vi "TDMS Advanced Append Multiple Headers.vi"   [LabVIEW 2023]
doc: "This example demonstrates how to append new header and raw data to an existing .tdms file using the Advanced TDMS VIs and functions. You can use the TDMS Advanced Asynchronous Read function to read the data from the .tdms file."
uses:
  <vilib>/Utility/TDMS File Viewer/NI_TDMS File Viewer.lvlib
panel:
  # "Overview: Demonstrates the use of the Advanced TDMS functions to append data with headers to a .tdms file.\nInstructions:\n1. Make sure you have already run TDMS Advanced Asynchronous Write.vi.\n2. Run this VI.\n3. Delete the TDMS file (located at [LabVIEW Data]\\Example TDMS Advanced Asynchronous Write.tdms) when you are done."
types:
  T1 = enum16{"open", "open or create", "create or replace", "create", "open (read-only)"}
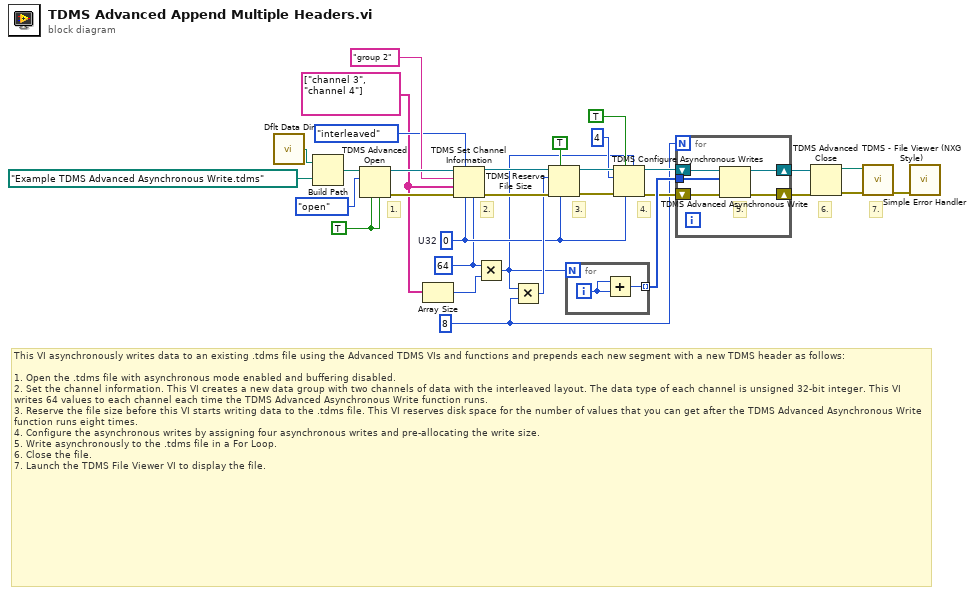
[diagram p0: block diagram]
diagram:
  w17 = TRUE ("enable asynchronous? (T)")
  w5 = 8 ("y")
  w3 = u32 64 ("samples per channel")
  w9 = u32 0  # U32
  w4 = string[] ["channel 3", "channel 4"] ("channel name(s)")
  # "4."
  # "This VI asynchronously writes data to an existing .tdms file using the Advanced TDMS VIs and functions and prepends each new segment with a new TDMS header as follows:\n\n1. Open the .tdms file with asynchronous mode enabled and buffering disabled.\n2. Set the channel information. This VI creates a new data group with two channels of data with the interleaved layout. The data type of each channel is unsigned 32-bit integer. This VI writes 64 values to each channel each time the TDMS Advanced Asynchronous Write function runs.\n3. Reserve the file size before this VI starts writing data to the .tdms file. This VI reserves disk space for the number of values that you can get after the TDMS Advanced Asynchronous Write function runs eight times.\n4. Configure the asynchronous writes by assigning four asynchronous writes and pre-allocating the write size.\n5. Write asynchronously to the .tdms file in a For Loop.\n6. Close the file.\n7. Launch the TDMS File Viewer VI to display the file."
  # "7."
  # "1."
  # "6."
  # "3."
  # "2."
  n1 = call <vilib>:"Dflt Data Dir.vi"() -> ("App:Default Data Directory"=w26:path)
  n2 = Build Path(base path=w26, name or relative path=path "Example TDMS Advanced Asynchronous Write.tdms") -> (appended path=w30:path)
  n3 = TDMS Advanced Open(4:w17, 6:w17, 10:T1."open" ("operation (0:open)"), 11:w30) -> (0:w28:errorcluster, 3:w27:refnum<k34>)  [unwired: 1 in, 1 out]
  n4 = Array Size(array=w4) -> (size(s)=w2:i32)
  n5 = TDMS Set Channel Information(4:w3, 6:w9, 7:enum16{"non-interleaved", "interleaved"}."interleaved" ("data layout (0:non-interleaved)"), 8:w28, 9:w4, 10:"group 2" ("group name (Untitled)"), 11:w27) -> (0:w20:errorcluster, 3:w19:refnum<k34>)
  n6 = Multiply(x=w3, y=w2) -> (x*y=w1:u32)
  n7 = Multiply(x=w1, y=w5) -> (x*y=w18:u32)
  n8 = TDMS Reserve File Size(6:w9, 7:TRUE ("append? (T)"), 8:w20, 10:w18, 11:w19) -> (0:w14:errorcluster, 3:w13:refnum<k34>)
  n9 = for {
    N: w1 -> [_]
    tunnel: [w32] -> w23 mode=indexing
    i -> [w33]
    n10 = Add(x=w33, y=w33) -> (x+y=w32:i32)
  }
  n11 = TDMS Configure Asynchronous Writes(5:w1, 6:w9, 7:TRUE ("pre-allocate? (F)"), 8:w14, 10:u32 4 ("number of buffers (4)"), 11:w13) -> (0:w11:errorcluster, 3:w12:refnum<k34>)  [unwired: 1 in]
  n12 = for {
    N: w5 -> [_]
    shift-right: [w35] -> w21
    shift-left: w12 -> [w37]
    shift-right: [w36] -> w22
    shift-left: w11 -> [w38]
    tunnel: w23 -> [w34]
    # "5."
    n13 = TDMS Advanced Asynchronous Write(8:w38, 10:w34, 11:w37) -> (0:w36:errorcluster, 3:w35:refnum<k34>)
  }
  n14 = TDMS Advanced Close(8:w22, 11:w21) -> (0:w16:errorcluster, 3:w15:path)  [unwired: 2 in]
  n15 = call <vilib>:"TDMS - File Viewer (NXG Style).vi"("error in"=w16, "file in"=w15) -> ("error out"=w6:errorcluster)  [unwired: 8 in, 1 out]
  n16 = call <vilib>:"Simple Error Handler.vi"("error in (no error)"=w6) -> ()  [unwired: 4 in, 5 out]
